vi "binary_gain_scheduler.vi"(8 "Binary scheduling constant":T2, 10 "Invert":bool, 11 "Error":dbl) -> (3 "Gains out":T1)   [LabVIEW 2011]
uses:
  gain_bin_sched_const.ctl
  gain_const.ctl
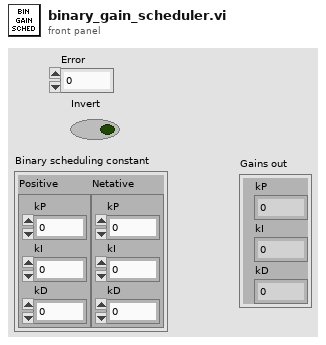
[diagram p1: front panel]
types:
  T1 = typedef "gain_const.ctl" = cluster{"kP":dbl, "kI":dbl, "kD":dbl}
  T2 = typedef "gain_bin_sched_const.ctl" = cluster{"Positive":cluster{"kP":dbl, "kI":dbl, "kD":dbl}, "Netative":cluster{"kP":dbl, "kI":dbl, "kD":dbl}}
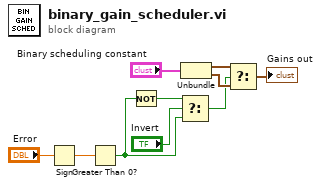
[diagram p0: block diagram]
diagram:
  n1 = Sign(1:"Error") -> (0:w9:dbl)
  n2 = Greater Than 0?(x=w9) -> (x > 0?=w6:bool)
  n3 = Not(x=w6) -> (.not. x?=w7:bool)
  n4 = Select(t=w7, s="Invert", f=w6) -> (s? t:f=w2:bool)
  n5 = Unbundle("Binary scheduling constant") -> ("Positive"=w4:cluster{"kP":dbl, "kI":dbl, "kD":dbl}, "Netative"=w3:cluster{"kP":dbl, "kI":dbl, "kD":dbl})
  n6 = Select(t=w4, s=w2, f=w3) -> (s? t:f=→"Gains out":cluster{"kP":dbl, "kI":dbl, "kD":dbl})
